vi "Acknowledge.vi"(7 "ack":refnum<k4>, 10 "parms in":T2={"subchannel"=0, "size (0)"=0, "abort (F)"=FALSE, "timeout"=-1, "ack id (0)"=0, "last elt? (F)"=FALSE, "valid? (T)"=FALSE, "GUID"=""}, 11 "messengerMbase in":refnum<class "MessengerMBase.lvclass">) -> (2 "parms out":T1, 3 "messengerMbase out":refnum<class "MessengerMBase.lvclass">)   [LabVIEW 2019, in "MessengerM.lvlib" / "MessengerMBase.lvclass"]
uses:
  <resource>/Channels/MessengerM/MessengerMBase/MessengerMBase.lvclass
  <resource>/Channels/MessengerM/ParmsIn.ctl
  <resource>/Channels/MessengerM/ParmsOut.ctl
  <resource>/Channels/MessengerM/MessengerMBase/MessengerMBase.lvclass/MessengerMBase.ctl
  <resource>/Channels/MessengerM/MessengerM.lvlib
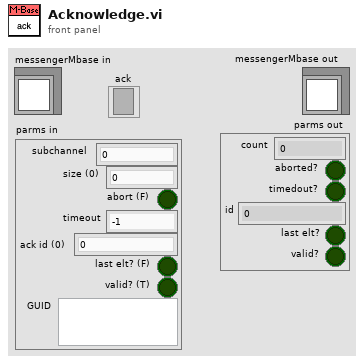
[diagram p1: front panel]
types:
  T1 = typedef "MessengerM.lvlib/ParmsOut.ctl" = cluster{"count":i32, "aborted?":bool, "timedout?":bool, "id":u32, "last elt?":bool, "valid?":bool}
  T2 = typedef "MessengerM.lvlib/ParmsIn.ctl" = cluster{"subchannel":i32, "size (0)":i32, "abort (F)":bool, "timeout":i32, "ack id (0)":u32, "last elt? (F)":bool, "valid? (T)":bool, "GUID":string}
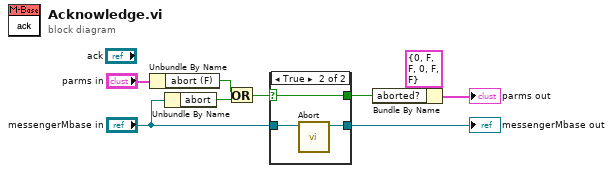
[diagram p0: block diagram]
diagram:
  n1 = Unbundle By Name("parms in") -> ("abort (F)"=w4:bool)
  n2 = Unbundle By Name("messengerMbase in") -> ("abort"=w8:bool)
  n3 = Or(x=w4, y=w8) -> (x .or. y?=w7:bool)
  n4 = case shown="True" w7 {
    selector: w7 -> [_ w13]
    tunnel: [w10 w11] -> w9
    tunnel: "messengerMbase in" -> [w10 w12]
    tunnel: [_ w13] -> w2
    frame False {
    }
    frame True {
      n5 = call-dynamic "Abort.vi"("messengerMbase in"=w12) -> ("messengerMbase out"=w11:refnum<class "MessengerMBase.lvclass">)  [unwired: 10 in]
    }
  }
  "messengerMbase out" <- w9
  n6 = Bundle By Name(cluster=T1 {"count"=0, "aborted?"=FALSE, "timedout?"=FALSE, "id"=0, "last elt?"=FALSE, "valid?"=FALSE} ("parms out"), "aborted?"=w2) -> (→"parms out":T1)
